vi "SVL Leq Sound Level (N Ch).vi"(6 "restart averaging (F)":bool, 8 "error in (no error)":errorcluster, 11 "scaled signals [EU]":waveform(dbl)[](array[waveform])) -> (0 "error out":errorcluster, 2 "unit labels":string[](array[string]), 3 "Leq sound levels [dB EU]":dbl[](array[numeric]) format="%.2f")   [LabVIEW 2017, in "SoundVib_SoundLevel.lvlib"]
doc: "Computes the linear averaged, or the equivalent continuous sound level (Leq), of <B>scaled signal [EU]</B>. <B>scaled signal [EU]</B> should have a zero DC component. You can attenuate the DC component with hardware AC-coupling filters and with software high-pass filters. Wire data to the <B>scaled signal [EU]</B> input to determine the polymorphic instance to use or manually select the instance."
uses:
  <vilib>/addons/Sound and Vibration/svt_Level/SoundVib_SoundLevel.lvlib
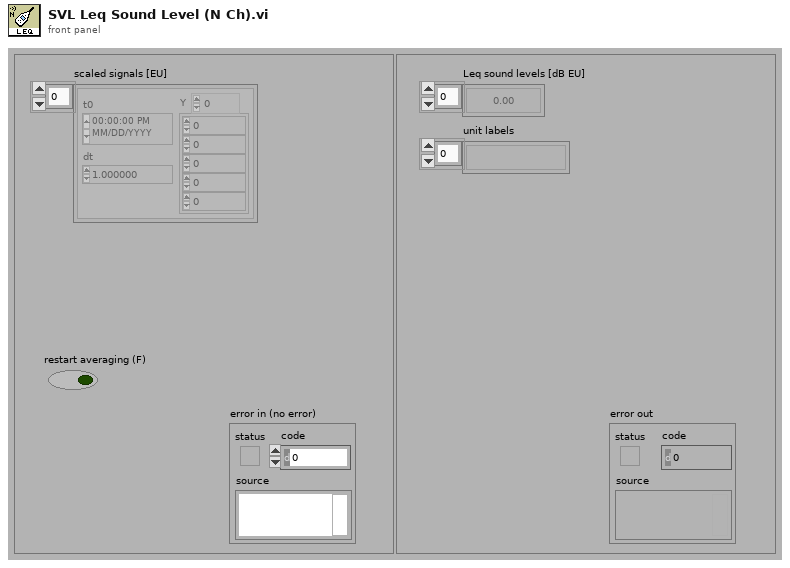
[diagram p1: front panel]
types:
  T1 = enum16{"RMS", "Running RMS", "Exp avg  ", "Dec exp avg ", "Peak", "Crest"}
  T2 = enum16{"Reset filter", "Restart averaging", "Continue processing"}
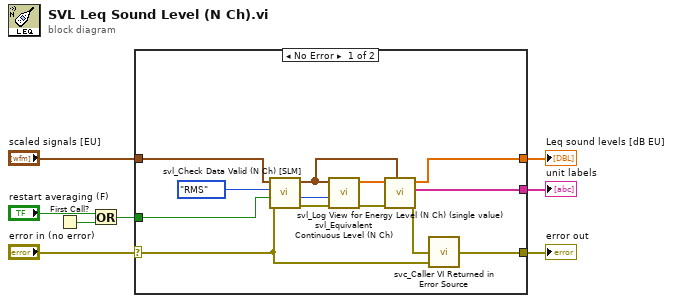
[diagram p0: block diagram]
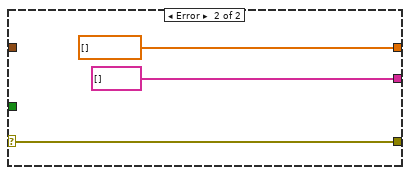
[diagram p2: hidden frame]
diagram:
  n1 = First Call?() -> (First Call?: T/F=w6:bool)
  n2 = Or(x="restart averaging (F)", y=w6) -> (x .or. y?=w4:bool)
  n3 = case shown="No Error" "error in (no error)" {
    selector: "error in (no error)" -> [w9 w24]
    tunnel: [w18 dbl[] [] ("energy levels [EU^2 rms]")] -> w8
    tunnel: [w17 string[] [] ("unit label [ ]")] -> w7
    tunnel: w4 -> [w13 _]
    tunnel: "scaled signals [EU]" -> [w10 _]
    tunnel: [w16 w24] -> w2
    frame No Error {
      n4 = call <vilib>:"svl_Check Data Valid (N Ch) [SLM].vi"("error in (no error)"=w9, "restart averaging (F)"=w13, "level analysis"=T1."RMS" ("Level Analysis"), "scaled signals [EU]"=w10) -> ("error out"=w15:errorcluster, "processing state"=w14:T2, "dup scaled signals [EU]"=w11:waveform(dbl)[])  [unwired: 5 in]
      n5 = call <vilib>:"svl_Equivalent Continuous Level (N Ch).vi"("error in (no error)"=w15, "processing state"=w14, "scaled signals [EU]"=w11) -> ("error out"=w20:errorcluster, "equivalent continuous levels [EU^2 rms]"=w19:dbl[])  [unwired: 7 in]
      n6 = call <vilib>:"svl_Log View for Energy Level (N Ch) (single value).vi"("waveform parameters"=w11, "error in (no error)"=w20, "energy levels [EU^2 rms]"=w19) -> ("error out"=w21:errorcluster, "unit label [ ]"=w17:string[], "energy levels [EU^2 rms]"=w18:dbl[])  [unwired: 6 in]
      n7 = call <vilib>:"svc_Caller VI Returned in Error Source.vi"("warning input to caller"=w9, "error in (no error)"=w21) -> ("error out"=w16:errorcluster)  [unwired: 3 in]
    }
    frame Error {
    }
  }
  "Leq sound levels [dB EU]" <- w8
  "unit labels" <- w7
  "error out" <- w2
